vi "Read Register.vi"(7 "Unit ID (A)":string="A", 8 "error in":errorcluster, 10 "Register address":u16, 11 "VISA Session In":refnum<visa-resource-name>="Alicat") -> (0 "error out":errorcluster, 2 "Register Value (I32)":i32, 3 "VISA Session Out":refnum<visa-resource-name>)   [LabVIEW 2018]
doc: "Reads the value of the specified register of an Alicat device."
uses:
  VISA Flush IO Buffer Mask.ctl
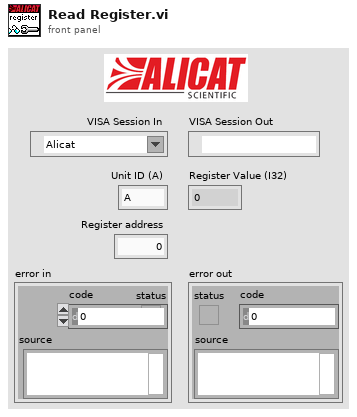
[diagram p1: front panel]
types:
  T1 = typedef "VISA Flush IO Buffer Mask.ctl" = u16
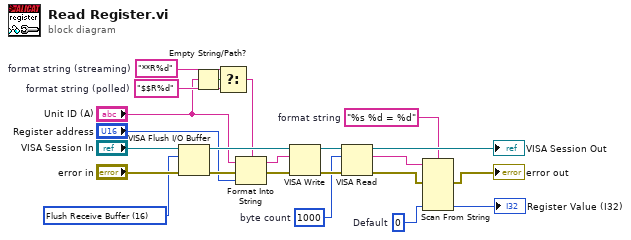
[diagram p0: block diagram]
diagram:
  w4 = "**R%d"  # format string (streaming)
  w8 = 0  # Default
  w6 = "$$R%d"  # format string (polled)
  w19 = T1 16 items=["Flush Receive Buffer"=16, "Write Transmit Buffer to Device"=32, "Flush Receive Buffer (No I/O)"=64, "Flush Transmit Buffer"=128] ("Mask")
  w12 = "%s %d = %d"  # format string
  w13 = u32 1000  # byte count
  n1 = VISA Flush I/O Buffer(VISA resource name="VISA Session In", mask (16)=w19, error in (no error)="error in") -> (VISA resource name out=w21:refnum<visa-resource-name>, error out=w10:errorcluster)
  n2 = Empty String/Path?(string/path="Unit ID (A)") -> (empty?=w5:bool)
  n3 = Select(t=w4, s=w5, f=w6) -> (s? t:f=w2:string)
  n4 = Format Into String(format string=w2, initial string="Unit ID (A)", error in=w10, "Register address") -> (resulting string=w11:string, error out=w9:errorcluster)
  n5 = VISA Write(VISA resource name=w21, write buffer=w11, error in (no error)=w9) -> (VISA resource name out=w18:refnum<visa-resource-name>, error out=w23:errorcluster)  [unwired: 1 out]
  n6 = VISA Read(VISA resource name=w18, byte count=w13, error in (no error)=w23) -> (VISA resource name out=→"VISA Session Out":refnum<visa-resource-name>, read buffer=w14:string, error out=w17:errorcluster)  [unwired: 1 out]
  n7 = Scan From String(format string=w12, input string=w14, error in=w17, default 3=w8) -> (error out=→"error out":errorcluster, output 3=→"Register Value (I32)":i32)  [unwired: 5 in, 2 out]
